vi "Read Client Handshake.vi"(8 "error in (no error)":errorcluster, 11 "Messaging Server Client in":refnum<class "Messaging Server Client.lvclass">) -> (0 "error out":errorcluster, 3 "Messaging Server Client out":refnum<class "Messaging Server Client.lvclass">)   [LabVIEW 2020, in "Volatus.lvlib" / "Messaging Server Client.lvclass"]
uses:
  Messaging Server Client.lvclass
  Messaging Server Client.lvclass/Messaging Server Client.ctl
  Volatus.lvlib
  lv-vecto/Vecto/proto/TcpClientHello/TcpClientHello.lvlib
  Module/Module.lvclass
  lv-vecto/Vecto/proto/ConnectStatus/Enumeration.ctl
  lv-vecto/Vecto/proto/ConnectStatus/ConnectStatus.lvlib
  VolatusAPI/VolatusAPI.lvclass
  C:/dev/lv20CE/relink/lv-volatus/Volatus/Module/Module.lvclass
  C:/dev/lv20CE/relink/lv-volatus/Volatus/Messaging Client/Messaging Server Client.lvclass
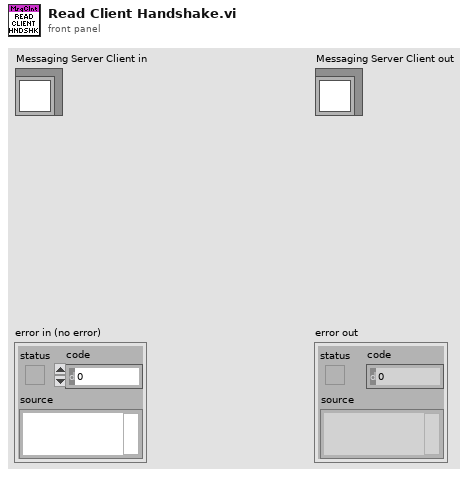
[diagram p1: front panel]
types:
  T1 = typedef "TcpClientHello.lvlib/Data.ctl" = cluster{"node_id":u32, "system":string, "cluster":string, "node_name":string, "app_version":string, "config_version":string, "config_hash":string, "node_alias":string}
  T2 = typedef "ConnectStatus.lvlib/Enumeration.ctl" = enum16{"STATUS_UNKNOWN", "STATUS_SUCCESS", "STATUS_ERROR", "STATUS_BAD_CONFIG", "STATUS_BAD_SYSTEM", "STATUS_BAD_CLUSTER", "STATUS_NOT_ALLOWED"}
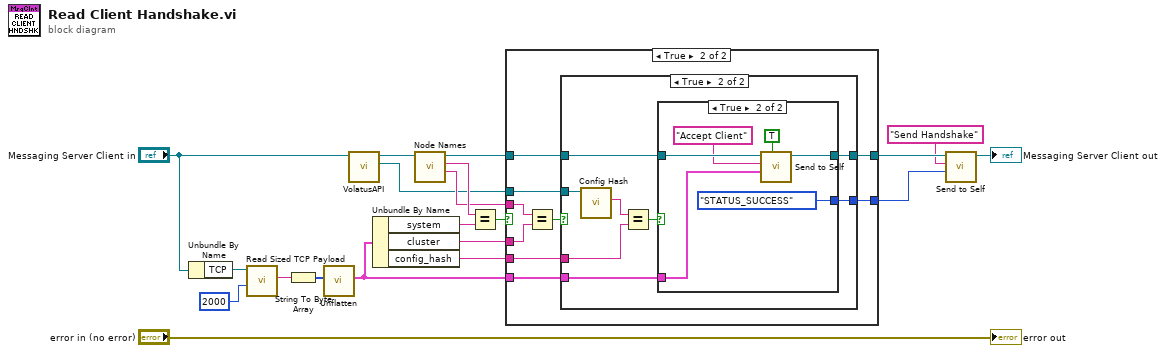
[diagram p0: block diagram]
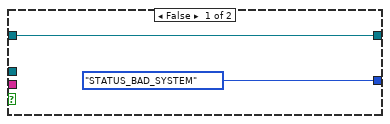
[diagram p2: hidden frame]
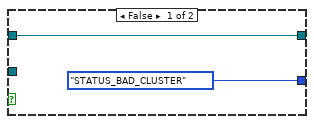
[diagram p3: hidden frame]
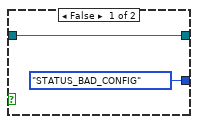
[diagram p4: hidden frame]
diagram:
  n1 = Unbundle By Name("Messaging Server Client in") -> ("TCP"=w18:refnum<k5>)
  n2 = call "Read Sized TCP Payload.vi"("timeout ms (100)"=2000, "TCP in"=w18) -> ("Payload"=w16:string)  [unwired: 7 in, 2 out]
  n3 = String To Byte Array(string=w16) -> (unsigned byte array=w15:u8[])
  n4 = call "Unflatten.vi"("Buffer"=w15) -> ("Data"=w5:T1)  [unwired: 9 in, 1 out]
  n5 = call "VolatusAPI.vi"("Module in"="Messaging Server Client in") -> ("VolatusAPI"=w8:refnum<class "VolatusAPI.lvclass">, "Module out"=w9:refnum<class "Messaging Server Client.lvclass">)  [unwired: 9 in]
  n6 = Unbundle By Name(w5) -> ("system"=w14:string, "cluster"=w10:string, "config_hash"=w6:string)
  n7 = call "Node Names.vi"("Module in"=w9) -> ("Cluster"=w11:string, "System"=w13:string, "Module out"=w7:refnum<class "Messaging Server Client.lvclass">)  [unwired: 6 in, 2 out]
  n8 = Equal?(x=w13, y=w14) -> (x = y?=w12:bool)
  n9 = case shown="True" w12 {
    tunnel: w11 -> [_ w31]
    tunnel: w10 -> [_ w27]
    tunnel: w8 -> [_ w29]
    tunnel: w7 -> [w22 w28]
    tunnel: w6 -> [_ w26]
    tunnel: w5 -> [_ w25]
    tunnel: [w22 w24] -> w2
    tunnel: [Enumeration."STATUS_BAD_SYSTEM" ("Handshake Status") w23] -> w3
    frame False {
    }
    frame True {
      n10 = Equal?(x=w31, y=w27) -> (x = y?=w30:bool)
      n11 = case shown="True" w30 {
        tunnel: w29 -> [_ w41]
        tunnel: w28 -> [w32 w37]
        tunnel: w26 -> [_ w39]
        tunnel: w25 -> [_ w36]
        tunnel: [w32 w35] -> w24
        tunnel: [Enumeration."STATUS_BAD_CLUSTER" ("Handshake Status") w34] -> w23
        frame False {
        }
        frame True {
          n12 = call "Config Hash.vi"("VolatusAPI in"=w41) -> ("Config Hash"=w40:string)  [unwired: 8 in, 2 out]
          n13 = Equal?(x=w40, y=w39) -> (x = y?=w38:bool)
          n14 = case shown="True" w38 {
            tunnel: w37 -> [w43 w48]
            tunnel: w36 -> [_ w44]
            tunnel: [w43 w47] -> w35
            tunnel: [Enumeration."STATUS_BAD_CONFIG" ("Handshake Status") Enumeration."STATUS_SUCCESS" ("Handshake Status")] -> w34
            frame False {
            }
            frame True {
              n15 = call "Send to Self.vi"("High Priority (F)"=TRUE, "Data"=w44, "Message ID"="Accept Client", "Module in"=w48) -> ("Module out"=w47:refnum<class "Messaging Server Client.lvclass">)  [unwired: 6 in, 1 out]
            }
          }
        }
      }
    }
  }
  n16 = call "Send to Self.vi"("Data"=w3, "Message ID"="Send Handshake", "Module in"=w2) -> ("Module out"=→"Messaging Server Client out":refnum<class "Messaging Server Client.lvclass">)  [unwired: 7 in, 1 out]
  "error out" <- "error in (no error)"
